vi "AlliGator Source Image ROI Storage [SGL] v3.vi"(7 "Current Source Image ROI Color":u32(colorbox), 8 "Error In":errorcluster, 9 "Current ROI Descriptor":T2 {"Contours"."Type" items=["No Selection", "Point", "Line", "Rectangle", "Oval", "Polygon", "Freehand Region", "Annulus", "Unused2", "Unused3", "Broken Line", "Freehand Line", "Rotated Rectangle"]}, 10 "Default Name (\"ROI\")":string="ROI", 11 "Action":T1=enum."Store New ROI") -> (0 "Error Out":errorcluster, 1 "Current ROI Descriptor":T2 {"Contours"."Type" items=["No Selection", "Point", "Line", "Rectangle", "Oval", "Polygon", "Freehand Region", "Annulus", "Unused2", "Unused3", "Broken Line", "Freehand Line", "Rotated Rectangle"]}, 2 "Current ROI Name":string, 3 "Current Source Image ROI Index":i32, 4 "Old ROI Name":string, 5 "Current Source Image ROI Color":u32(colorbox), 6 "Message":string)   [LabVIEW 2021, in "AlliGator ROIs.lvlib"]
doc: "Handles single Source Image ROI storage."
uses:
  AlliGator ROIs.lvlib
  AlliGator ROI Manager Actions.ctl
  Globals, Variables, Constants/AlliGator Variables List.ctl
  Image/Named ROI Description.ctl
  ee07913d-caa1-4b3a-856f-a30c4ade46b3.vi
  Variant/Variant to Data/Variant to I32.vi
  GUI/GUI.lvlib
  Image/Image.lvlib
  Globals, Variables, Constants/AlliGator Globals, Variables & Constants.lvlib
  Variant/Variant to Data/Variant to Data.lvlib
  Strings/Strings.lvlib
panel:
  # "see the AlliGator License on the block diagram (Ctrl+E or Window:Show Block Diagram)"
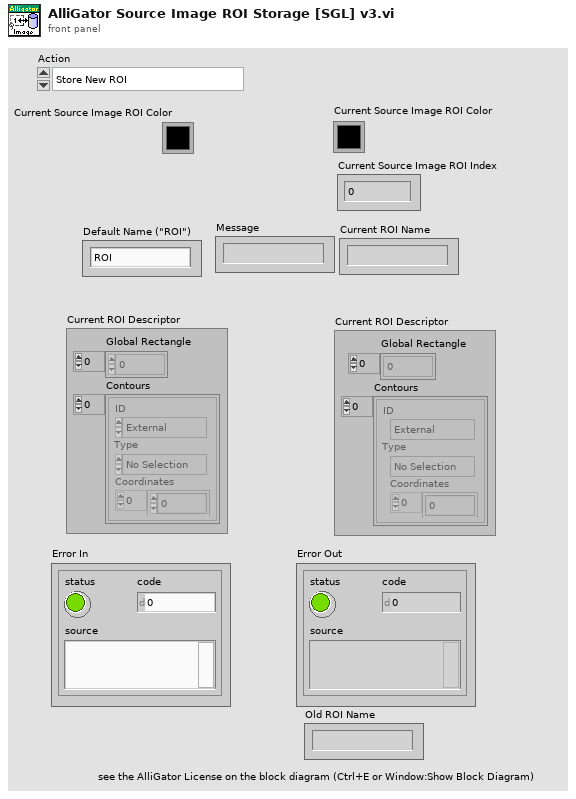
[diagram p1: front panel]
types:
  T1 = typedef "AlliGator ROIs.lvlib/AlliGator ROI Manager Actions.ctl" = enum16{"Undefined", "Delete Current ROI", "Delete All Unselected ROIs", "Delete Multiple ROIs", "Delete All ROIs", "Swap ROIs", "Insert ROI", "Update Current ROI Descriptor", "Rename Current ROI", "Store New ROI", "Store Multiple ROIs", "Select Next ROI", "Select Previous ROI", "Find Selected ROI", "Show All ROIs", "Update ROI Manager Window", "Merge All ROIs", "Unmerge ROI", "Set Selected ROI by ID"}
  T2 = typedef "ROI Descriptor" = cluster{"Global Rectangle":i32[], "Contours":cluster{"ID":enum32{"External", "Internal"}, "Type":u32, "Coordinates":i32[]}[]}
  T3 = typedef "AlliGator Globals, Variables & Constants.lvlib/AlliGator Variables List.ctl" = enum16{"---- GUI ----", "GUI:Initialization Status", "GUI:State Indicators Refnum", "GUI:Original AlliGator Menu Items", "GUI:Current Action Loop State", "GUI:Script in progress", "GUI:Playback", "GUI:Loop Playback", "GUI:Search ROI Used", "GUI:Search ROI", "Decay Graph Max Legend Size", "Intensity Graph Max Legend Size", "Decay Statistics Graph Max Legend Size", "Phasor Graph Max Legend Size", "Phasor Ratio Graph Max Legend Size", "Lifetime Graph Max Legend Size", "---- Files ----", "Files:Export Dataset Frames as Individual Files", "Files:Show Batch Export Help Balloons", "Files:Frames in Dataset", "Files:ptu File Frame Start Indices", "Files:Current Frame in Dataset", "Files:Current Frame Timestamp", "Files:Dataset Loaded", "Files:Dataset Metadata", "Files:Dataset Channel", "Files:Dataset Data Description", "Files:Background Dataset Metadata", "Files:Background Dataset Channel", "Files:Background Dataset Data Description", "Files:Background File Subtraction", "Files:Background File Path", "Files:Background File Pile-up Correction", "Files:Background File Pixel Well Capacity", "Files:Background File Scaling Factor", "Files:Current Dataset Load Settings", "Files:Dataset Path", "Files:ICCD-specific Information", "Files:Macrotime Gate Separation", "------ Python Plugins ------", "Python Plugins:Information", "Python Plugins:Python Session", "Python Plugins:Valid Python Session?", "---- Source Image ----", "Source Image:ROIs", "Source Image:Current ROI", "Source Image:ROI Event Refnum", "X_Source Image Display Range", "X_Source Image Palette Information", "X_Type of Displayed Image", "X_Time Gate Slider", "Source Image:Palette List", "Source Image:Scale", "Source Image:ROI Overlay Color", "Source Image:Overlay to Erase", "Source Image:Is Displayed Image Accumulated", "Source Image:White Light Image Modified", "Source Image:Mask Image Modified", "---- Image Profile Window ----", "Image Profile:Window Event Refnum", "Image Profile:IntensityType", "Image Profile:Intensity Average Type", "Image Profile:Intensity-weighted SDV", "Image Profile:Box Profile Type", "Image Profile:Window Open", "Image Profile:Plotted Fit Parameter", "------ Phasor Graph -------", "Phasor Graph:Show Line", "---- Phasor Plot ---", "Phasor Plot:Parameters Changed", "Phasor Plot:FLI Dataset Modified since last Calculation", "Phasor Harmonics Data", "Selected Phasor Harmonics", "Phasor Harmonic Manager Event Refnum", "Phasor Plot:ROIs", "Phasor Plot:Current ROI", "Phasor Plot:ROI Event Refnum", "Phasor Plot:Image Reference Points", "Phasor Plot:Computed", "Phasor Plot:Palette Information", "Phasor Plot:Palette List", "Phasor Plot:Phasor Ratio Palette Information", "Phasor Plot:Phasor Ratio Palette List", "Phasor Plot:Image Scale", "Phasor Plot:Image Overlay to Erase", "Phasor Plot:Image Elements to Update", "Phasor Plot:Current Calculation Parameters", "Phasor Plot:Current Calibration Options", "Phasor Plot:Reset Cumulated Phasor Plot", "Phasor Plot:Reference 1", "Phasor Plot:Lifetime Reference 1", "Phasor Plot:Reference 1 Frequency", "Phasor Plot:Reference 2", "Phasor Plot:Lifetime Reference 2", "Phasor Plot:Reference 2 Frequency", "---- Decay Analysis ----", "Number of Selected Decays to Fit", "LS Fit Results", "LAR Fit Results", "BS Fit Results", "Last Decay Max - Min", "Best Fit Parameters", "Best Fit Parameter Names", "Actual Size X", "Actual Size Y", "Binning X", "Binning Y", "Actual # Gates", "Dataset Number", "Gates to...", "Gates Skipped", "Gates to keep", "Gate Step", "Gate Separation", "Reversed Gates", "Pile-up Correction", "Pixel Well Capacity", "Background Subtracted", "Background Subtraction Method", "Background Definition Range", "Background File (deprecated)", "Number of Dataset Accumulated", "Array of Accumulated Dataset Paths", "Do Averaged Datasets", "Destination File Path", "Process Plot Target", "Use 1/D as Phasor Frequency", "---- Decay Fit Parameter Map -----", "Decay Fit Parameter Map:Palette Information", "Decay Fit Parameter Map:Palette List", "---- Parameter Map ----", "Parameter Map:Palette Information", "Parameter Map:Palette List", "------- Local Decay Window ---------", "Local Decay Graph Window:Event Refnum", "Local Decay Graph Window:Use normalized IRF for convolution", "----- Miscellaneous ----", "Misc:Skippable Dialog Windows Status"}
  T4 = typedef "Image.lvlib/Named ROI Description.ctl" = cluster{"ROI Descriptor":T2, "ROI Name":string, "Overlay Color":u32}
  T5 = typedef "AlliGator ROIs.lvlib/AlliGator Image ROI Event refnum.ctl" = refnum<user-event>
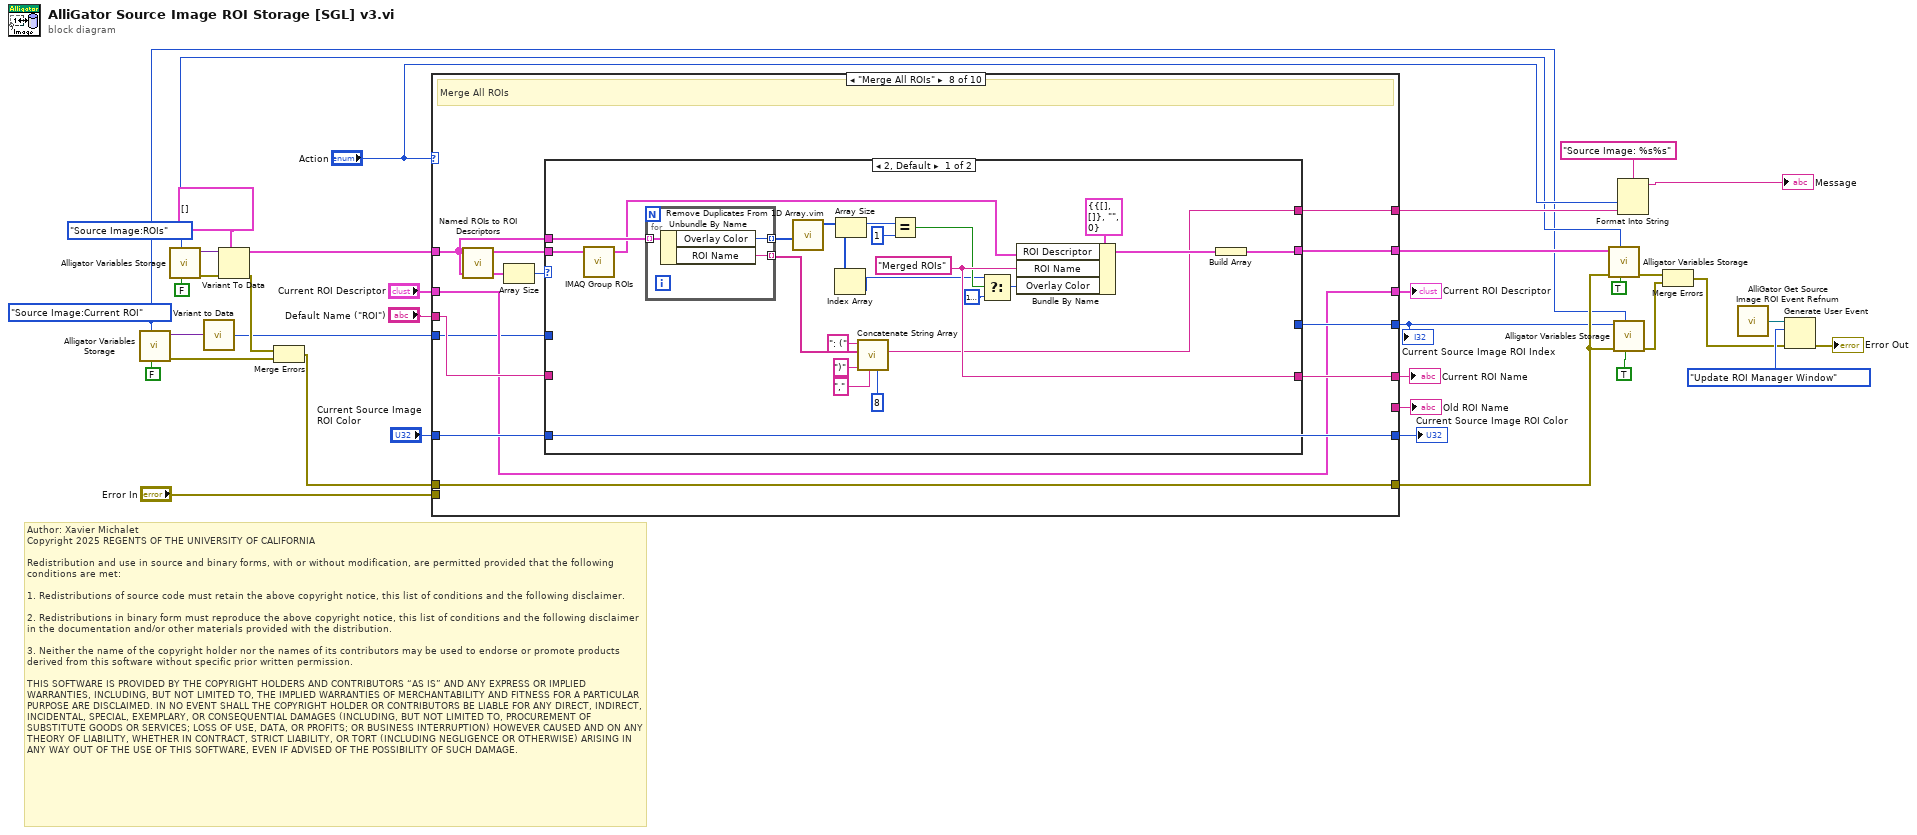
[diagram p0: block diagram]
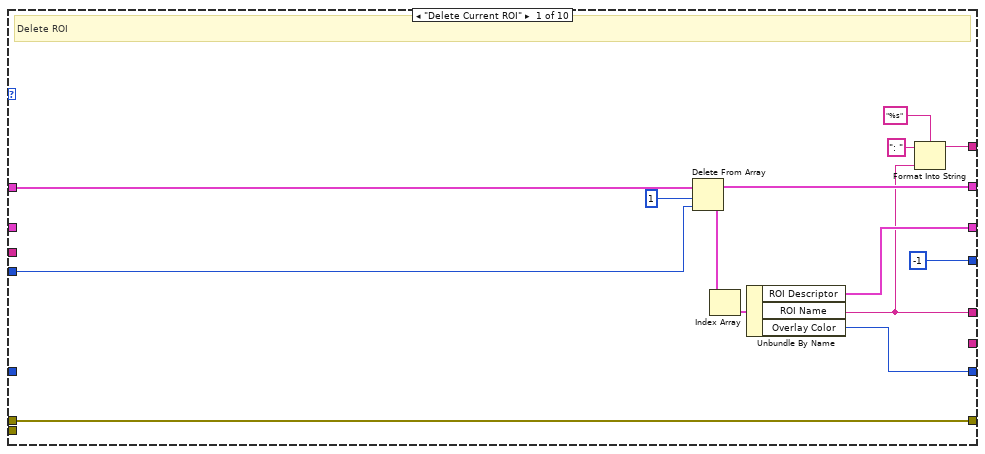
[diagram p2: hidden frame]
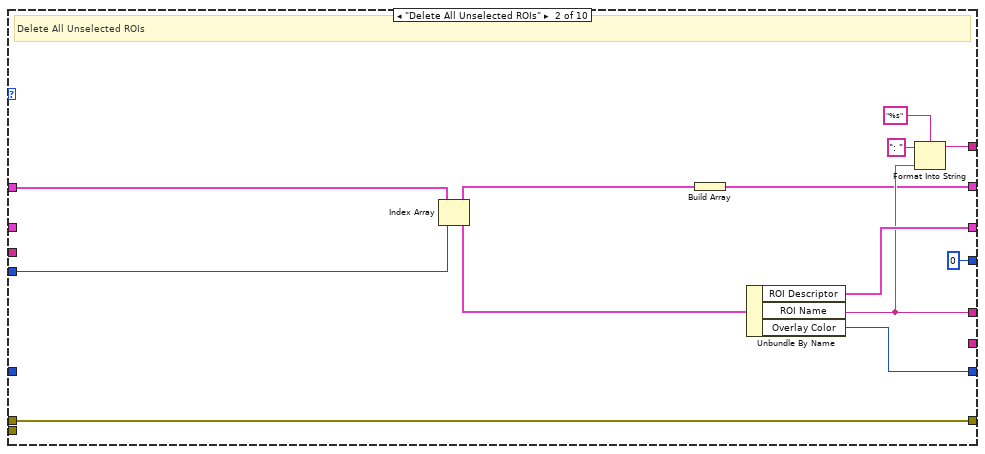
[diagram p3: hidden frame]
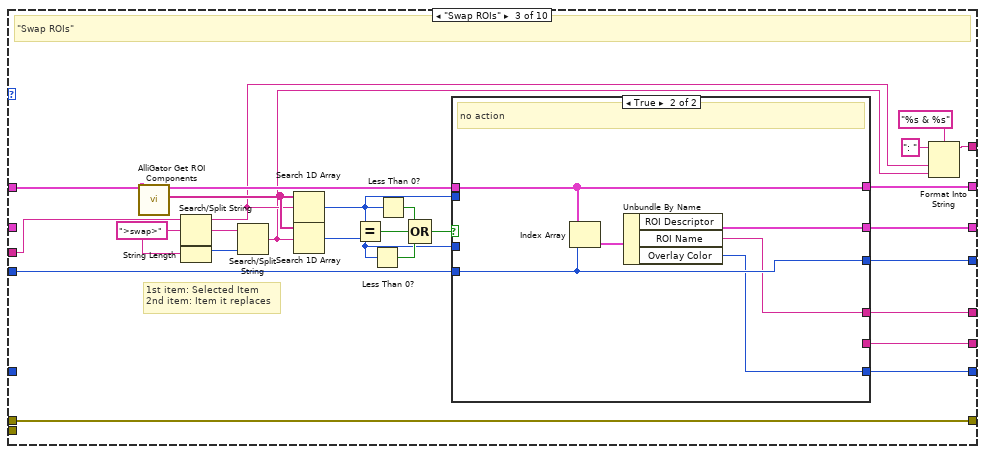
[diagram p4: hidden frame]
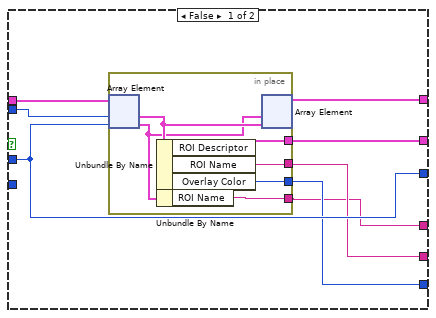
[diagram p5: hidden frame]
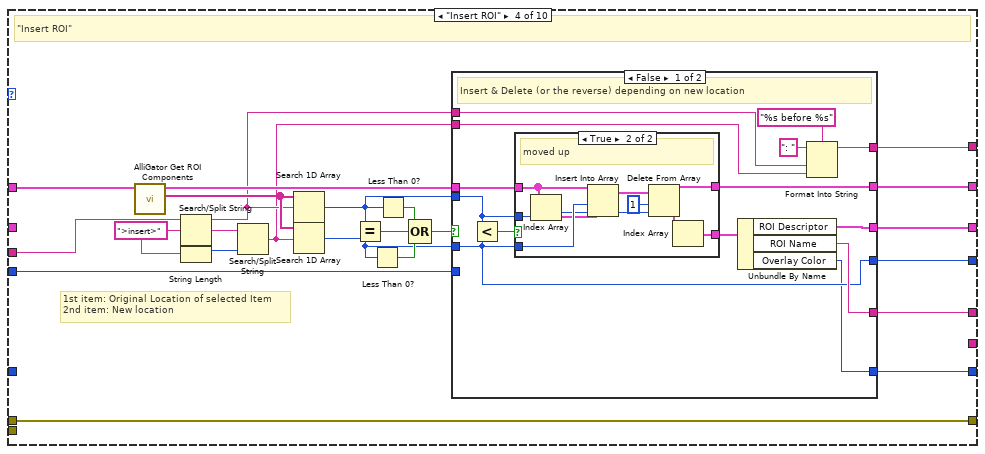
[diagram p6: hidden frame]
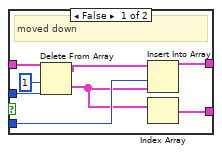
[diagram p7: hidden frame]
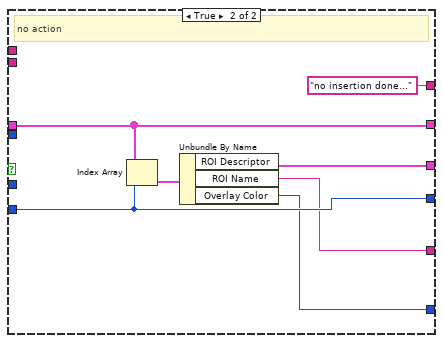
[diagram p8: hidden frame]
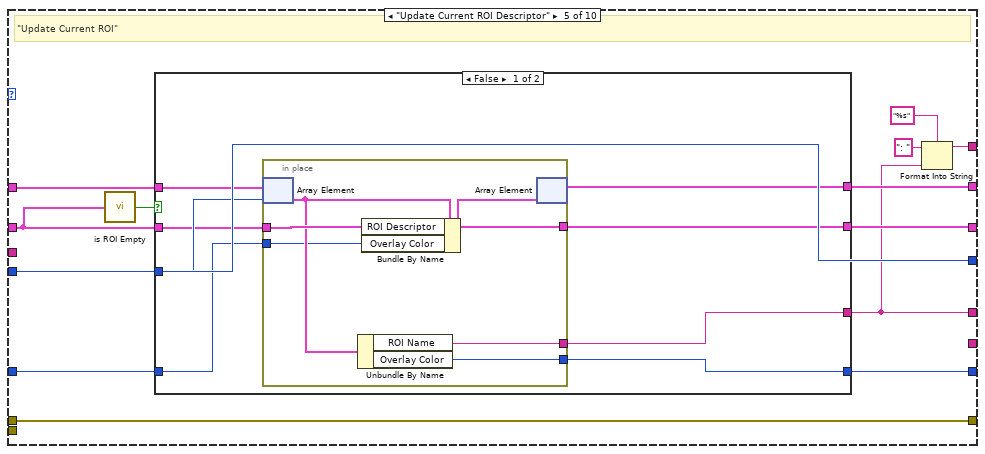
[diagram p9: hidden frame]
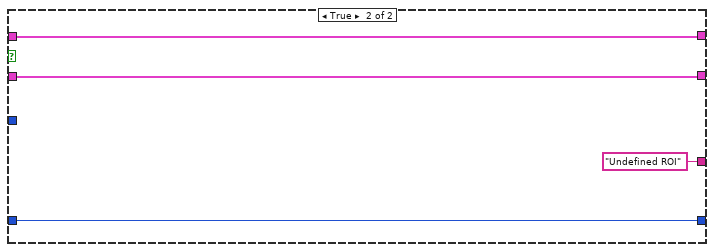
[diagram p10: hidden frame]
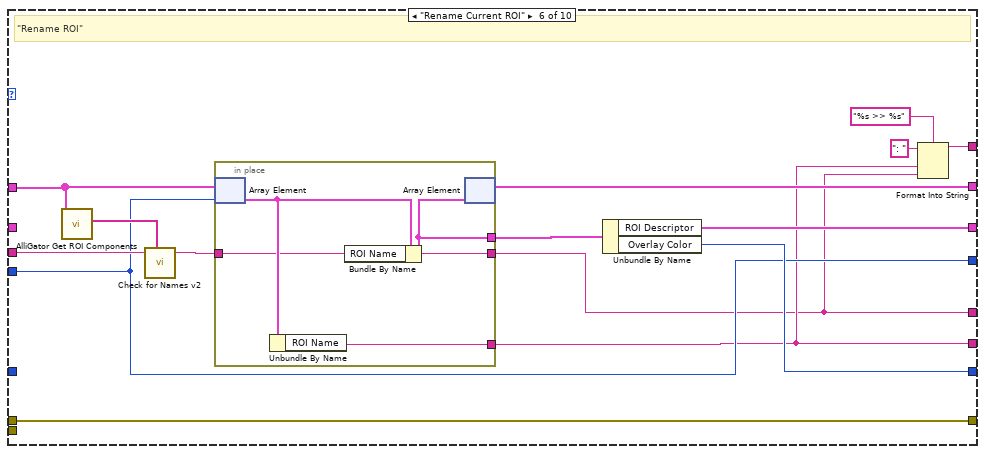
[diagram p11: hidden frame]
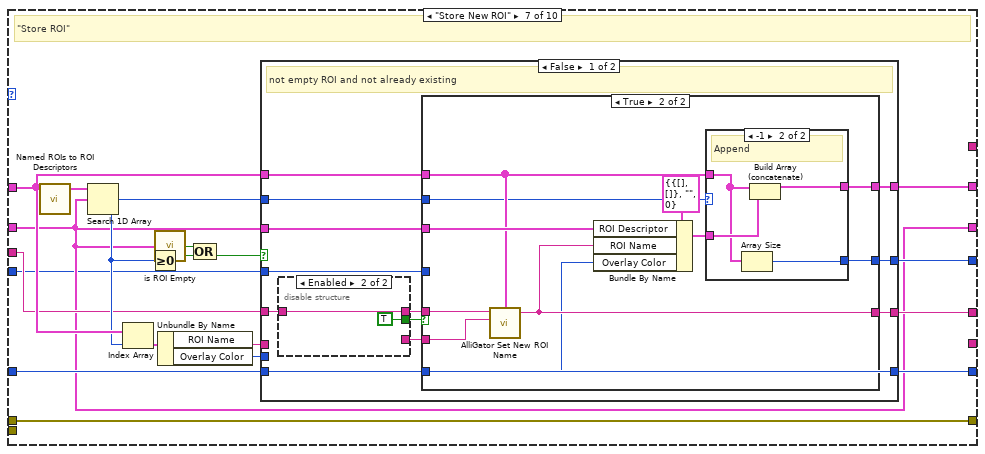
[diagram p12: hidden frame]
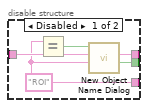
[diagram p13: hidden frame]
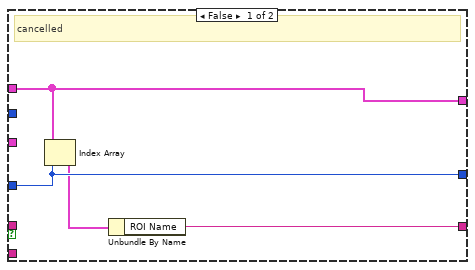
[diagram p14: hidden frame]
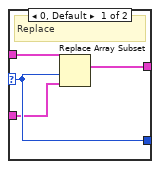
[diagram p15: hidden frame]
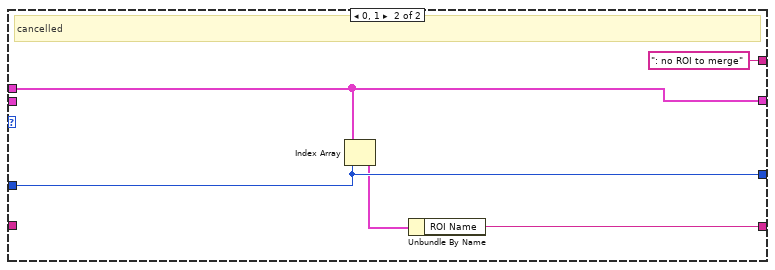
[diagram p17: hidden frame]
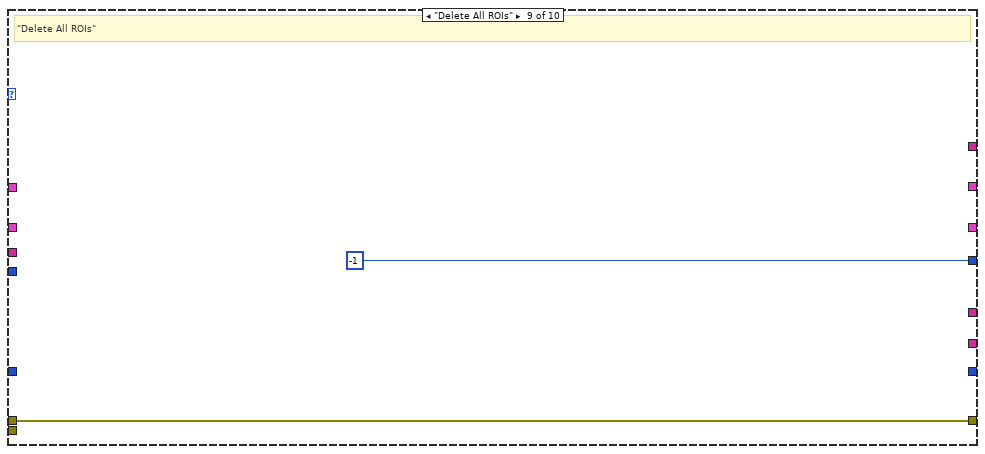
[diagram p18: hidden frame]
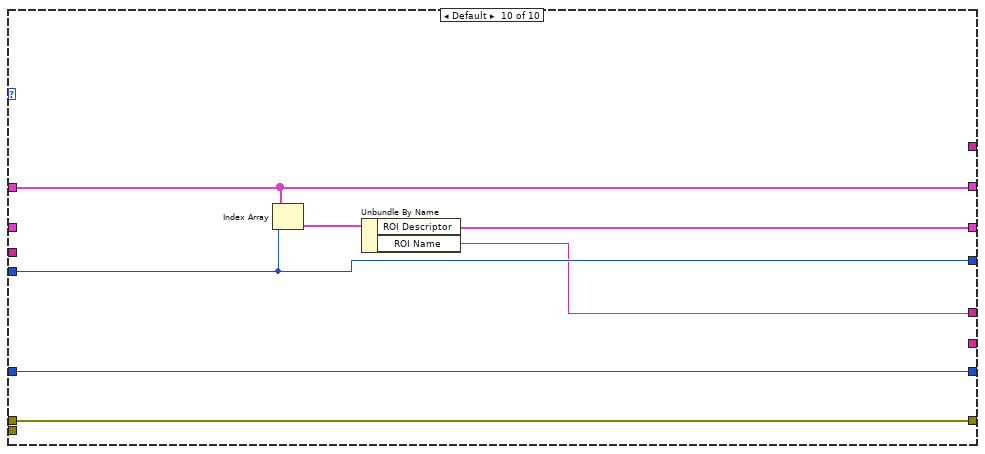
[diagram p19: hidden frame]
diagram:
  w1 = AlliGator_Variables_List."Source Image:Current ROI" ("Alligator Variable")
  w2 = AlliGator_Variables_List."Source Image:ROIs" ("Alligator Variable")
  # "Author: Xavier Michalet\nCopyright 2025 REGENTS OF THE UNIVERSITY OF CALIFORNIA\n\nRedistribution and use in source and binary forms, with or without modification, are permitted provided that the following conditions are met:\n\n1. Redistributions of source code must retain the above copyright notice, this list of conditions and the following disclaimer.\n\n2. Redistributions in binary form must reproduce the above copyright notice, this list of conditions and the following disclaimer in the documentation and/or other materials provided with the distribution.\n\n3. Neither the name of the copyright holder nor the names of its contributors may be used to endorse or promote products derived from this software without specific prior written permission.\n\nTHIS SOFTWARE IS PROVIDED BY THE COPYRIGHT HOLDERS AND CONTRIBUTORS “AS IS” AND ANY EXPRESS OR IMPLIED WARRANTIES, INCLUDING, BUT NOT LIMITED TO, THE IMPLIED WARRANTIES OF MERCHANTABILITY AND FITNESS FOR A PARTICULAR PURPOSE ARE DISCLAIMED. IN NO EVENT SHALL THE COPYRIGHT HOLDER OR CONTRIBUTORS BE LIABLE FOR ANY DIRECT, INDIRECT, INCIDENTAL, SPECIAL, EXEMPLARY, OR CONSEQUENTIAL DAMAGES (INCLUDING, BUT NOT LIMITED TO, PROCUREMENT OF SUBSTITUTE GOODS OR SERVICES; LOSS OF USE, DATA, OR PROFITS; OR BUSINESS INTERRUPTION) HOWEVER CAUSED AND ON ANY THEORY OF LIABILITY, WHETHER IN CONTRACT, STRICT LIABILITY, OR TORT (INCLUDING NEGLIGENCE OR OTHERWISE) ARISING IN ANY WAY OUT OF THE USE OF THIS SOFTWARE, EVEN IF ADVISED OF THE POSSIBILITY OF SUCH DAMAGE."
  n1 = call "Alligator Variables Storage.vi"("Get(F)/Set"=FALSE, "AlliGator Variable"=w1) -> ("Error Out"=w28:errorcluster, "Data out"=w31:variant)  [unwired: 7 in, 1 out]
  n2 = call "Alligator Variables Storage.vi"("Get(F)/Set"=FALSE, "AlliGator Variable"=w2) -> ("Error Out"=w35:errorcluster, "Data out"=w36:variant)  [unwired: 7 in, 1 out]
  n3 = call-poly "Variant to Data.vi"("Variant"=w31) -> ("Value"=w22:i32)  [unwired: 8 in]
  n4 = Variant To Data(error in=w35, type=T4[] [] ("Stored ROIs in"), Variant=w36) -> (data=w23:T4[], error out=w27:errorcluster)
  n5 = Merge Errors(w27, w28) -> (w8:errorcluster)
  n6 = case shown="\"Merge All ROIs\"" "Action" {
    tunnel: w23 -> [w50 w56 w69 w112 w180 w209 w232 w285 _ w329]
    tunnel: w22 -> [w49 w53 w87 w129 w177 w205 w219 w287 _ w328]
    tunnel: [w47 w55 w86 w128 w179 w206 w235 w293 _ w329] -> w19
    tunnel: [-1 ("Current ROI out") 0 ("Value") w85 w127 w177 w205 w234 w292 -1 ("index of element") w328] -> w3
    tunnel: "Current ROI Descriptor" -> [_ _ _ _ w176 _ w220 w288 _ _]
    tunnel: [w42 w61 w74 w117 w178 w213 w220 w288 _ w326] -> w18
    tunnel: "Default Name (\"ROI\")" -> [_ _ w83 w126 _ w210 w227 w291 _ _]
    tunnel: [w40 w59 w73 w116 w169 w200 w224 w290 _ w325] -> w17
    tunnel: [_ _ w84 _ _ w201 _ _ _ _] -> w16
    tunnel: [w43 w62 w70 w113 w174 w212 w223 w289 _ w331] -> w15
    tunnel: "Current Source Image ROI Color" -> [_ _ _ _ w173 _ w221 w289 _ w331]
    tunnel: [w41 w60 w67 w111 w171 w202 _ w283 _ _] -> w9
    tunnel: w8 -> [w37 w52 w63 w108 w168 w199 w218 w282 w323 w330]
    tunnel: "Error In" -> [_ _ _ _ _ _ _ _ _ _]
    tunnel: [w37 w52 w63 w108 w168 w199 w218 w282 w323 w330] -> w6
    frame "Delete Current ROI" {
      # "Delete ROI"
      n7 = Delete From Array(array=w50, length=1, index=w49) -> (deleted portion=w45:T4[], array with subset deleted=w47:T4[])
      n8 = Index Array(array=w45) -> (element=w44:T4)  [unwired: 1 in]
      n9 = Unbundle By Name(w44) -> ("ROI Descriptor"=w42:T2, "ROI Name"=w40:string, "Overlay Color"=w43:u32)
      n10 = Format Into String(format string="%s", initial string=": ", w40) -> (resulting string=w41:string)  [unwired: 1 in, 1 out]
    }
    frame "Delete All Unselected ROIs" {
      # "Delete All Unselected ROIs"
      n11 = Index Array(array=w56, index=w53) -> (element=w54:T4)
      n12 = Build Array(w54) -> (w55:T4[])
      n13 = Unbundle By Name(w54) -> ("ROI Descriptor"=w61:T2, "ROI Name"=w59:string, "Overlay Color"=w62:u32)
      n14 = Format Into String(format string="%s", initial string=": ", w59) -> (resulting string=w60:string)  [unwired: 1 in, 1 out]
    }
    frame "Swap ROIs" {
      w81 = ">swap>" ("search string/char (-)")
      # "1st item: Selected Item\n2nd item: Item it replaces"
      # "\"Swap ROIs\""
      n15 = call "AlliGator Get ROI Components.vi"("Stored ROIs"=w69) -> ("ROI Names"=w79:string[])  [unwired: 8 in, 2 out]
      n16 = Search/Split String(string=w83, search string/char (-)=w81) -> (substring before match=w65:string, match + rest of string=w82:string)  [unwired: 1 in, 1 out]
      n17 = String Length(string=w81) -> (length=w80:i32)
      n18 = Search/Split String(string=w82, offset (0)=w80) -> (match + rest of string=w64:string)  [unwired: 1 in, 2 out]
      n19 = Search 1D Array(1D array=w79, element=w65) -> (index of element=w72:i32)  [unwired: 1 in]
      n20 = Search 1D Array(1D array=w79, element=w64) -> (index of element=w71:i32)  [unwired: 1 in]
      n21 = Equal?(x=w72, y=w71) -> (x = y?=w76:bool)
      n22 = Less Than 0?(x=w71) -> (x < 0?=w77:bool)
      n23 = Less Than 0?(x=w72) -> (x < 0?=w78:bool)
      n24 = Compound Arithmetic op=OR(w78, w76, w77) -> (w75:bool)
      n25 = case shown="True" w75 {
        tunnel: w87 -> [_ w106]
        tunnel: [w94 w107] -> w86
        tunnel: [w91 w106] -> w85
        tunnel: [w89 _] -> w84
        tunnel: w69 -> [w95 w107]
        tunnel: [w92 w104] -> w74
        tunnel: [w88 w103] -> w73
        tunnel: w72 -> [w93 _]
        tunnel: w71 -> [w91 _]
        tunnel: [w90 w102] -> w70
        frame False {
          n26 = in-place {
            in-place-border: [w100] -> w92
            in-place-border: [w99] -> w89
            in-place-border: [w98] -> w90
            in-place-border: [w96] -> w88
            n27 = in-place-array #1(w95, w93, w91) -> (w101:T4, w97:T4)
            n28 = Unbundle By Name(w101) -> ("ROI Descriptor"=w100:T2, "ROI Name"=w99:string, "Overlay Color"=w98:u32)
            n29 = Unbundle By Name(w97) -> ("ROI Name"=w96:string)
            n30 = in-place-array #1(w97, w101) -> (w94:T4[])  [unwired: 2 out]
          }
        }
        frame True {
          # "no action"
          n31 = Index Array(array=w107, index=w106) -> (element=w105:T4)
          n32 = Unbundle By Name(w105) -> ("ROI Descriptor"=w104:T2, "ROI Name"=w103:string, "Overlay Color"=w102:u32)
        }
      }
      n33 = Format Into String(format string="%s & %s", initial string=": ", w65, w64) -> (resulting string=w67:string)  [unwired: 1 in, 1 out]
    }
    frame "Insert ROI" {
      w124 = ">insert>" ("search string/char (-)")
      # "1st item: Original Location of selected Item\n2nd item: New location"
      # "\"Insert ROI\""
      n34 = call "AlliGator Get ROI Components.vi"("Stored ROIs"=w112) -> ("ROI Names"=w122:string[])  [unwired: 8 in, 2 out]
      n35 = Search/Split String(string=w126, search string/char (-)=w124) -> (substring before match=w110:string, match + rest of string=w125:string)  [unwired: 1 in, 1 out]
      n36 = String Length(string=w124) -> (length=w123:i32)
      n37 = Search/Split String(string=w125, offset (0)=w123) -> (match + rest of string=w109:string)  [unwired: 1 in, 2 out]
      n38 = Search 1D Array(1D array=w122, element=w110) -> (index of element=w115:i32)  [unwired: 1 in]
      n39 = Search 1D Array(1D array=w122, element=w109) -> (index of element=w114:i32)  [unwired: 1 in]
      n40 = Equal?(x=w115, y=w114) -> (x = y?=w119:bool)
      n41 = Less Than 0?(x=w114) -> (x < 0?=w120:bool)
      n42 = Less Than 0?(x=w115) -> (x < 0?=w121:bool)
      n43 = Compound Arithmetic op=OR(w121, w119, w120) -> (w118:bool)
      n44 = case shown="False" w118 {
        tunnel: w129 -> [_ w166]
        tunnel: [w140 w167] -> w128
        tunnel: [w136 w166] -> w127
        tunnel: w112 -> [w142 w167]
        tunnel: [w138 w164] -> w117
        tunnel: [w137 w163] -> w116
        tunnel: w115 -> [w141 _]
        tunnel: w114 -> [w136 _]
        tunnel: [w135 w162] -> w113
        tunnel: [w133 "no insertion done..."] -> w111
        tunnel: w110 -> [w131 _]
        tunnel: w109 -> [w130 _]
        frame False {
          # "Insert & Delete (or the reverse) depending on new location"
          n45 = Less?(x=w141, y=w136) -> (x < y?=w143:bool)
          n46 = case shown="True" w143 {
            tunnel: w142 -> [w151 w160]
            tunnel: w141 -> [w150 w156]
            tunnel: w136 -> [w146 w159]
            tunnel: [w147 w154] -> w140
            tunnel: [w144 w152] -> w139
            frame False {
              # "moved down"
              n47 = Delete From Array(array=w151, length=1, index=w150) -> (deleted portion=w145:T4[], array with subset deleted=w148:T4[])
              n48 = Insert Into Array(array=w148, index=w146, new element=w145) -> (w147:T4[])
              n49 = Index Array(array=w145) -> (element=w144:T4)  [unwired: 1 in]
            }
            frame True {
              # "moved up"
              n50 = Index Array(array=w160, index=w156) -> (element=w158:T4)
              n51 = Insert Into Array(array=w160, index=w159, new element=w158) -> (w157:T4[])
              n52 = Delete From Array(array=w157, length=1, index=w156) -> (deleted portion=w153:T4[], array with subset deleted=w154:T4[])
              n53 = Index Array(array=w153) -> (element=w152:T4)  [unwired: 1 in]
            }
          }
          n54 = Unbundle By Name(w139) -> ("ROI Descriptor"=w138:T2, "ROI Name"=w137:string, "Overlay Color"=w135:u32)
          n55 = Format Into String(format string="%s before %s", initial string=": ", w131, w130) -> (resulting string=w133:string)  [unwired: 1 in, 1 out]
        }
        frame True {
          # "no action"
          n56 = Index Array(array=w167, index=w166) -> (element=w165:T4)
          n57 = Unbundle By Name(w165) -> ("ROI Descriptor"=w164:T2, "ROI Name"=w163:string, "Overlay Color"=w162:u32)
        }
      }
    }
    frame "Update Current ROI Descriptor" {
      # "\"Update Current ROI\""
      n58 = call "is ROI Empty.vi"("Current ROI Descriptor"=w176) -> ("Empty ROI?"=w175:bool)  [unwired: 8 in]
      n59 = case shown="False" w175 {
        tunnel: w180 -> [w188 w198]
        tunnel: [w187 w198] -> w179
        tunnel: [w186 w197] -> w178
        tunnel: [w185 "Undefined ROI" ("ROI Name")] -> w169
        tunnel: w177 -> [w184 _]
        tunnel: w176 -> [w183 w197]
        tunnel: [w182 w195] -> w174
        tunnel: w173 -> [w181 w195]
        frame False {
          n60 = in-place {
            in-place-border: w183 -> [w193]
            in-place-border: [w193] -> w186
            in-place-border: [w191] -> w185
            in-place-border: [w190] -> w182
            in-place-border: w181 -> [w189]
            n61 = in-place-array #2(w188, w184) -> (w192:T4)
            n62 = Unbundle By Name(w192) -> ("ROI Name"=w191:string, "Overlay Color"=w190:u32)
            n63 = Bundle By Name(cluster=w192, "ROI Descriptor"=w193, "Overlay Color"=w189) -> (w194:T4)
            n64 = in-place-array #2(w194) -> (w187:T4[])  [unwired: 1 out]
          }
        }
        frame True {
        }
      }
      n65 = Format Into String(format string="%s", initial string=": ", w169) -> (resulting string=w171:string)  [unwired: 1 in, 1 out]
    }
    frame "Rename Current ROI" {
      # "\"Rename ROI\""
      n66 = call "AlliGator Get ROI Components.vi"("Stored ROIs"=w209) -> ("ROI Names"=w211:string[])  [unwired: 8 in, 2 out]
      n67 = call "Check for Names v2.vi"("New Name"=w210, "Name List"=w211) -> ("New Name"=w208:string)  [unwired: 4 in, 3 out]
      n68 = in-place {
        in-place-border: w208 -> [w214]
        in-place-border: [w217] -> w207
        in-place-border: [w215] -> w201
        in-place-border: [w214] -> w200
        n69 = in-place-array #3(w209, w205) -> (w216:T4)
        n70 = Unbundle By Name(w216) -> ("ROI Name"=w215:string)
        n71 = Bundle By Name(cluster=w216, "ROI Name"=w214) -> (w217:T4)
        n72 = in-place-array #3(w217) -> (w206:T4[])  [unwired: 1 out]
      }
      n73 = Unbundle By Name(w207) -> ("ROI Descriptor"=w213:T2, "Overlay Color"=w212:u32)
      n74 = Format Into String(format string="%s >> %s", initial string=": ", w201, w200) -> (resulting string=w202:string)  [unwired: 1 in, 1 out]
    }
    frame "Store New ROI" {
      # "\"Store ROI\""
      n75 = call "Named ROIs to ROI Descriptors.vi"("Named ROIs"=w232) -> ("ROI Descriptors"=w233:T2[])  [unwired: 10 in]
      n76 = Search 1D Array(1D array=w233, element=w220) -> (index of element=w229:i32)  [unwired: 1 in]
      n77 = Index Array(array=w232, index=w229) -> (element=w231:T4)
      n78 = Greater Or Equal To 0?(x=w229) -> (x >= 0?=w228:bool)
      n79 = call "is ROI Empty.vi"("Current ROI Descriptor"=w220) -> ("Empty ROI?"=w225:bool)  [unwired: 8 in]
      n80 = Unbundle By Name(w231) -> ("ROI Name"=w230:string, "Overlay Color"=w222:u32)
      n81 = Compound Arithmetic op=OR(w225, w228) -> (w226:bool)
      n82 = case shown="False" w226 {
        tunnel: [w247 w281] -> w235
        tunnel: [w246 w279] -> w234
        tunnel: w220 -> [w245 _]
        tunnel: w232 -> [w244 w281]
        tunnel: w230 -> [_ w280]
        tunnel: w229 -> [w243 w279]
        tunnel: w227 -> [w240 _]
        tunnel: [w241 w280] -> w224
        tunnel: [w239 w278] -> w223
        tunnel: w222 -> [_ w278]
        tunnel: w221 -> [w239 _]
        tunnel: w219 -> [w236 _]
        frame False {
          # "not empty ROI and not already existing"
          n83 = disable-structure shown="Enabled" {
            disable-tunnel: [w252 w254] -> w242
            disable-tunnel: w240 -> [w250 w254]
            disable-tunnel: [w249 _] -> w238
            disable-tunnel: [w248 TRUE ("OK")] -> w237
            frame Disabled {
              w249 = "ROI" ("x")
              n84 = Equal?(x=w249, y=w250) -> (x = y?=w251:bool)
              n85 = call "New Object Name Dialog.vi"("String Name (\"object\")"=w249, "Object Name in"=w250, "Enable"=w251) -> ("OK"=w248:bool, "Object Name out"=w252:string)  [unwired: 6 in, 1 out]
            }
            frame Enabled {
            }
          }
          n86 = case shown="True" w237 {
            tunnel: [w257 w269] -> w247
            tunnel: [w258 w268] -> w246
            tunnel: w245 -> [_ w265]
            tunnel: w244 -> [w257 w264]
            tunnel: w243 -> [_ w263]
            tunnel: w242 -> [_ w262]
            tunnel: [w255 w261] -> w241
            tunnel: w239 -> [_ w260]
            tunnel: w238 -> [_ w259]
            tunnel: w236 -> [w258 _]
            frame False {
              # "cancelled"
              n87 = Index Array(array=w257, index=w258) -> (element=w256:T4)
              n88 = Unbundle By Name(w256) -> ("ROI Name"=w255:string)
            }
            frame True {
              n89 = call "AlliGator Set New ROI Name.vi"("Stored ROIs in"=w264, "ROI Name in"=w262, "Default Name (\"\")"=w259) -> ("ROI Name out"=w261:string)  [unwired: 6 in]
              n90 = Bundle By Name(cluster=T4 {"ROI Descriptor"={"Global Rectangle"=[], "Contours"=[]}, "ROI Name"="", "Overlay Color"=0} ("Named ROI Description"), "ROI Descriptor"=w265, "ROI Name"=w261, "Overlay Color"=w260) -> (w266:T4)
              n91 = case shown="-1" w263 {
                selector: w263 -> [w272 _]
                tunnel: [w271 w277] -> w269
                tunnel: [w272 w276] -> w268
                tunnel: w266 -> [w270 w275]
                tunnel: w264 -> [w273 w274]
                frame 0, Default {
                  # "Replace"
                  n92 = Replace Array Subset(array=w273, new element=w270, index=w272) -> (w271:T4[])
                }
                frame -1 {
                  # "Append"
                  n93 = Array Size(array=w274) -> (size(s)=w276:i32)
                  n94 = Build Array (concatenate)(w274, w275) -> (w277:T4[])
                }
              }
            }
          }
        }
        frame True {
          # "no need to change or empty ROI"
        }
      }
    }
    frame "Merge All ROIs" {
      # "Merge All ROIs"
      n95 = call "Named ROIs to ROI Descriptors.vi"("Named ROIs"=w285) -> ("ROI Descriptors"=w286:T2[])  [unwired: 10 in]
      n96 = Array Size(array=w285) -> (size(s)=w284:i32)
      n97 = case shown="2, Default" w284 {
        tunnel: [w311 w321] -> w293
        tunnel: [_ w322] -> w292
        tunnel: w285 -> [w310 w321]
        tunnel: w291 -> [_ _]
        tunnel: [w313 w319] -> w290
        tunnel: w289 -> [_ _]
        tunnel: w287 -> [_ w322]
        tunnel: w286 -> [w301 _]
        tunnel: [w294 ": no ROI to merge" ("Formatted String")] -> w283
        frame 2, Default {
          w313 = "Merged ROIs" ("ROI Name")
          n98 = call "IMAQ Group ROIs"("ROI Descriptors"=w301) -> ("ROI Descriptor out"=w300:T2)  [unwired: 3 in, 1 out]
          n99 = for {
            tunnel: w310 -> [w317] mode=indexing
            tunnel: [w316] -> w309 mode=indexing
            tunnel: [w315] -> w299 mode=indexing
            n100 = Unbundle By Name(w317) -> ("Overlay Color"=w316:u32, "ROI Name"=w315:string)
          }
          n101 = call "Remove Duplicates From 1D Array.vim"("array"=w309) -> ("array with duplicates removed"=w305:u32[])  [unwired: 10 in]
          n102 = Index Array(array=w305) -> (element=w304:u32)  [unwired: 1 in]
          n103 = Array Size(array=w305) -> (size(s)=w308:i32)
          n104 = call "Concatenate String Array.vi"("Max Number of Elements (None: -1)"=8, "Separator (TAB)"=",", "Suffix (\"\")"=")" ("Suffix (\"\")"), "String Array"=w299, "Prefix (\"\")"=": (" ("Prefix (\"\")")) -> ("Formatted String"=w294:string)  [unwired: 6 in]
          n105 = Equal?(x=w308, y=1) -> (x = y?=w306:bool)
          n106 = Select(t=w304, s=w306, f=u32 16777216) -> (s? t:f=w303:u32)
          n107 = Bundle By Name(cluster=T4 {"ROI Descriptor"={"Global Rectangle"=[], "Contours"=[]}, "ROI Name"="", "Overlay Color"=0} ("Named ROI Description"), "ROI Descriptor"=w300, "ROI Name"=w313, "Overlay Color"=w303) -> (w312:T4)
          n108 = Build Array(w312) -> (w311:T4[])
        }
        frame 0, 1 {
          # "cancelled"
          n109 = Index Array(array=w321, index=w322) -> (element=w320:T4)
          n110 = Unbundle By Name(w320) -> ("ROI Name"=w319:string)
        }
      }
    }
    frame "Delete All ROIs" {
      # "\"Delete All ROIs\""
    }
    frame Default {
      n111 = Index Array(array=w329, index=w328) -> (element=w327:T4)
      n112 = Unbundle By Name(w327) -> ("ROI Descriptor"=w326:T2, "ROI Name"=w325:string)
    }
  }
  "Current ROI Descriptor" <- w18
  "Current Source Image ROI Index" <- w3
  "Current ROI Name" <- w17
  "Old ROI Name" <- w16
  "Current Source Image ROI Color" <- w15
  n113 = call "Alligator Variables Storage.vi"("Get(F)/Set"=TRUE, "AlliGator Variable"=w2, "Error In"=w6, "Data in"=w19) -> ("Error Out"=w25:errorcluster)  [unwired: 5 in, 2 out]
  n114 = call "Alligator Variables Storage.vi"("Get(F)/Set"=TRUE, "AlliGator Variable"=w1, "Error In"=w6, "Data in"=w3) -> ("Error Out"=w26:errorcluster)  [unwired: 5 in, 2 out]
  n115 = Format Into String(format string="Source Image: %s%s", "Action", w9) -> (resulting string=→"Message":string)  [unwired: 2 in, 1 out]
  n116 = Merge Errors(w25, w26) -> (w4:errorcluster)
  n117 = call "AlliGator Get Source Image ROI Event Refnum.vi"() -> ("Source Image ROI Event Refnum"=w12:T5)
  n118 = Generate User Event(user event=w12, event data cluster=AlliGator_ROI_Manager_Actions."Update ROI Manager Window" ("event data"), error in=w4) -> (error out=→"Error Out":errorcluster)  [unwired: 1 in, 1 out]
